vi "Word_Set_Chart_Scale.vi"(0 "Word.InlineShapes":refnum<k7>, 1 "gridlines":T1, 5 "Type":i32(ring)=1 items=["xlCategory"=1, "xlSeriesAxis"=3, "xlValue"=2], 9 "Chart index":i16=-1, 11 "error in":errorcluster, 12 "axis config":T2={"autoscale"=FALSE, "min"=0.0, "max"=0.0, "scale type"=-4132} {"scale type" items=["xlScaleLinear"=-4132, "xlScaleLogarithmic"=-4133]; "max" format="%.2f"; "min" format="%.2f"}) -> (15 "error out":errorcluster)   [LabVIEW 2010, in "NI_ReportGenerationToolkit.lvlib"]
uses:
  <vilib>/addons/_office/NI_ReportGenerationToolkit.lvlib
panel:
  in  "Graph.Axes":refnum<k7>
  in  "Graph.Chart":refnum<k7>
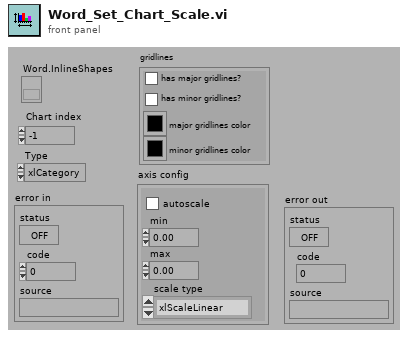
[diagram p1: front panel]
types:
  T1 = cluster{"has major gridlines?":bool, "has minor gridlines?":bool, "major gridlines color":u32, "minor gridlines color":u32}
  T2 = cluster{"autoscale":bool, "min":dbl, "max":dbl, "scale type":i32}
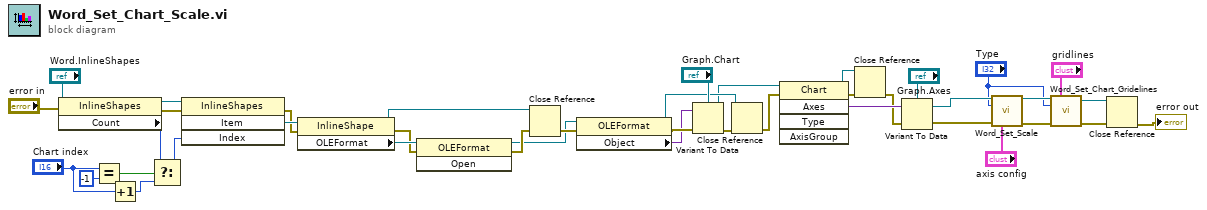
[diagram p0: block diagram]
diagram:
  n1 = property class="InlineShapes"(reference="Word.InlineShapes", error in="error in") -> (reference out=w21:refnum<k7>, error out=w39:errorcluster, "Count"=w16:i32)
  n2 = Equal?(x="Chart index", y=i16 -1) -> (x = y?=w20:bool)
  n3 = Increment(x="Chart index") -> (x+1=w18:i16)
  n4 = Select(t=w16, s=w20, f=w18) -> (s? t:f=w15:i32)
  n5 = invoke class="InlineShapes" method="Item"(reference=w21, error in=w39, "Index"=w15) -> (error out=w26:errorcluster, "Item"=w31:refnum<k7>)  [unwired: 1 in, 2 out]
  n6 = property class="InlineShape"(reference=w31, error in=w26) -> (reference out=w34:refnum<k7>, error out=w3:errorcluster, "OLEFormat"=w4:refnum<k7>)
  n7 = invoke class="OLEFormat" method="Open"(reference=w4, error in=w3) -> (reference out=w1:refnum<k7>, error out=w2:errorcluster)  [unwired: 1 in, 1 out]
  n8 = Close Reference(reference=w34, error in (no error)=w2) -> (error out=w33:errorcluster)
  n9 = property class="OLEFormat"(reference=w1, error in=w33) -> (reference out=w32:refnum<k7>, error out=w38:errorcluster, "Object"=w37:variant)
  n10 = Variant To Data(error in=w38, Variant=w37, type="Graph.Chart") -> (error out=w35:errorcluster, data=w30:refnum<k7>)
  n11 = Close Reference(reference=w32, error in (no error)=w35) -> (error out=w27:errorcluster)
  n12 = invoke class="Chart" method="Axes"(reference=w30, error in=w27) -> (reference out=w8:refnum<k7>, error out=w9:errorcluster, "Axes"=w29:variant)  [unwired: 3 in, 2 out]
  n13 = Close Reference(reference=w8, error in (no error)=w9) -> (error out=w23:errorcluster)
  n14 = Variant To Data(error in=w23, Variant=w29, type="Graph.Axes") -> (error out=w25:errorcluster, data=w24:refnum<k7>)
  n15 = call <vilib>:"Word_Set_Scale.vi"("Axes in"=w24, "Type"="Type", "error in"=w25, "axis config"="axis config") -> ("Axes out"=w12:refnum<k7>, "error out"=w13:errorcluster)  [unwired: 5 in, 5 out]
  n16 = call <vilib>:"Word_Set_Chart_Gridelines.vi"("Axes in"=w12, "gridlines"="gridlines", "Type"="Type", "error in"=w13) -> ("Axes out"=w6:refnum<k7>, "error out"=w7:errorcluster)  [unwired: 10 out]
  n17 = Close Reference(reference=w6, error in (no error)=w7) -> (error out=→"error out":errorcluster)
